vi "DetectTriggerGivenTrack.vi"(8 "error in (no error)":errorcluster, 9 "CameraFrame":i32, 10 "Track":T1, 11 "TriggerOnTurnsTwoColors in":refnum<class "TriggerOnTurnsTwoColors.lvclass">) -> (0 "error out":errorcluster, 2 "Triggered?":bool, 3 "TriggerOnTurnsTwoColors out":refnum<class "TriggerOnTurnsTwoColors.lvclass">)   [LabVIEW 2019, in "TriggerOnTurnsTwoColors.lvclass"]
uses:
  TriggerOnTurnsTwoColors.lvclass
  WormTrackCluster.ctl
  StimulusObject.lvclass
  TrackTerminationReasonEnum.ctl
  TriggerOnTurnsTwoColors.lvclass/TriggerOnTurnsTwoColors.ctl
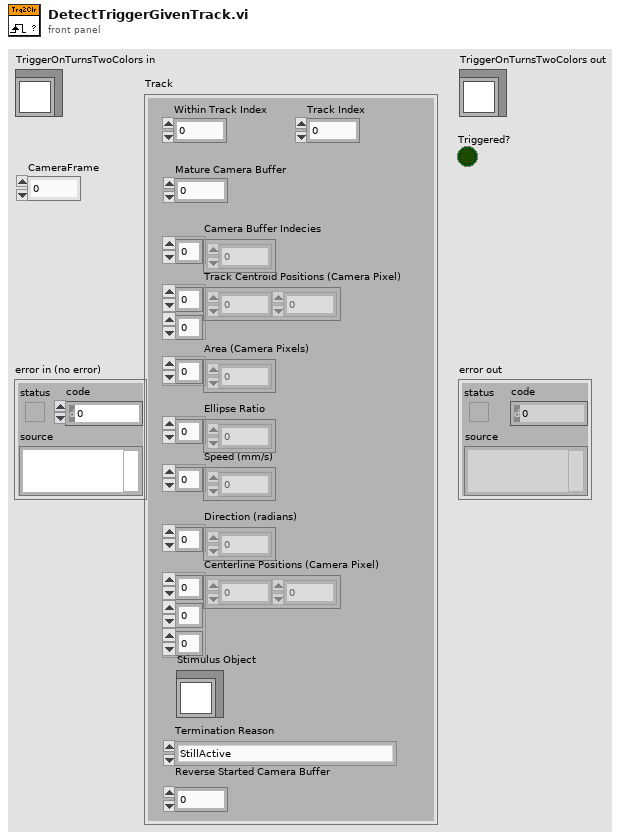
[diagram p1: front panel]
types:
  T1 = typedef "WormTrackCluster.ctl" = cluster{"Track Centroid Positions (Camera Pixel)":sgl[][], "Within Track Index":i32, "Camera Buffer Indecies":i32[], "Area (Camera Pixels)":i32[], "Speed (mm/s)":sgl[], "Direction (radians)":sgl[], "Centerline Positions (Camera Pixel)":sgl[][][], "Ellipse Ratio":sgl[], "Stimulus Object":refnum<class "StimulusObject.lvclass">, "Termination Reason":T2, "Track Index":i32, "Mature Camera Buffer":i32, "Reverse Started Camera Buffer":i32}
  T2 = typedef "TrackTerminationReasonEnum.ctl" = enum16{"StillActive", "MaxDisplacement", "NoBlobsLeft", "AreaIncrease", "AreaDecrease", "ExperimentEnded"}
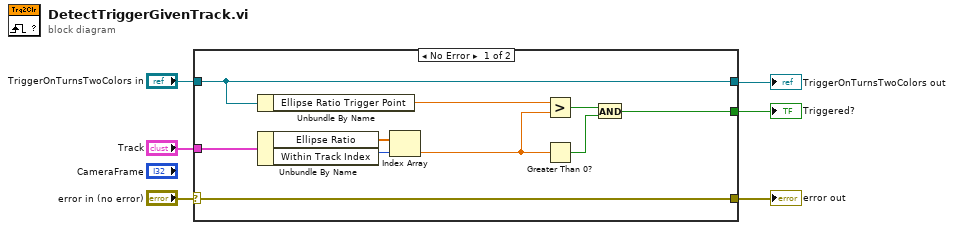
[diagram p0: block diagram]
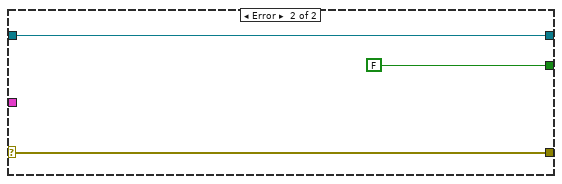
[diagram p2: hidden frame]
diagram:
  n1 = case shown="No Error" "error in (no error)" {
    selector: "error in (no error)" -> [w16 w19]
    tunnel: [w16 w19] -> w3
    tunnel: "TriggerOnTurnsTwoColors in" -> [w9 w18]
    tunnel: [w9 w18] -> w6
    tunnel: "Track" -> [w15 _]
    tunnel: [w8 FALSE] -> w4
    frame No Error {
      n2 = Unbundle By Name(w9) -> ("Ellipse Ratio Trigger Point"=w12:sgl)
      n3 = Unbundle By Name(w15) -> ("Ellipse Ratio"=w14:sgl[], "Within Track Index"=w13:i32)
      n4 = Index Array(array=w14, index=w13) -> (element=w7:sgl)
      n5 = Greater?(x=w12, y=w7) -> (0:w11:bool)
      n6 = Greater Than 0?(x=w7) -> (x > 0?=w10:bool)
      n7 = And(x=w11, y=w10) -> (x .and. y?=w8:bool)
    }
    frame Error {
    }
  }
  "error out" <- w3
  "TriggerOnTurnsTwoColors out" <- w6
  "Triggered?" <- w4
